vi "Straighten.vi"(6 "Go":bool, 8 "LockedHeading":dbl, 9 "Yaw":dbl, 10 "RightIn":dbl, 11 "LeftIn":dbl) -> (1 "Complete":bool, 2 "RightOut":dbl, 3 "LeftOut":dbl)   [LabVIEW 2015]
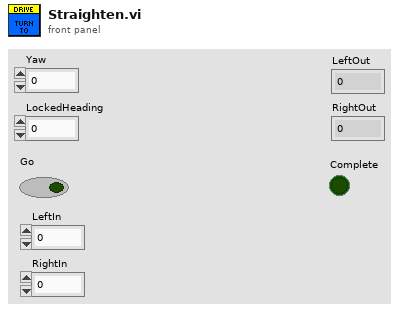
[diagram p1: front panel]
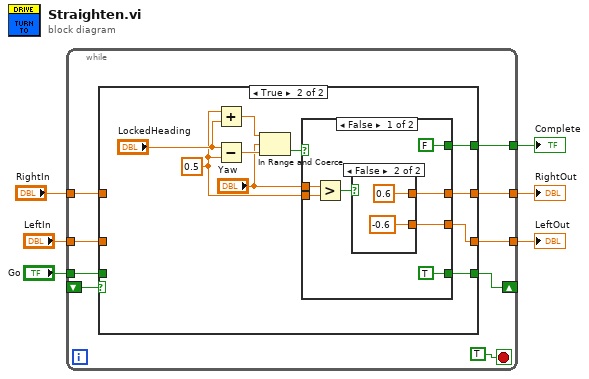
[diagram p0: block diagram]
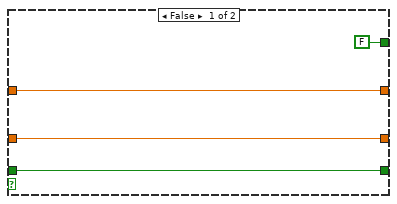
[diagram p2: hidden frame]
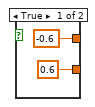
[diagram p3: hidden frame]
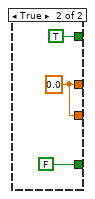
[diagram p4: hidden frame]
diagram:
  n1 = while {
    tunnel: "Go" -> [w15]
    shift-right: [w14] -> _
    shift-left: _ -> [w13]
    tunnel: "LeftIn" -> [w12]
    tunnel: [w11] -> w1
    tunnel: "RightIn" -> [w10]
    tunnel: [w9] -> w2
    tunnel: [w8] -> w3
    stop <- TRUE stop-if-true
    n2 = case shown="True" w13 {
      tunnel: [w19 w21] -> w14
      tunnel: w15 -> [w19 _]
      tunnel: [w18 w23] -> w11
      tunnel: w12 -> [w18 _]
      tunnel: [w17 w22] -> w9
      tunnel: w10 -> [w17 _]
      tunnel: [FALSE w20] -> w8
      frame False {
      }
      frame True {
        w25 = 0.5 ("y")
        n3 = Add(x=w25, y="LockedHeading") -> (x+y=w28:dbl)
        n4 = Subtract(x="LockedHeading", y=w25) -> (x-y=w27:dbl)
        n5 = In Range and Coerce(upper limit=w28, x="Yaw", lower limit=w27) -> (In Range?=w29:bool)  [unwired: 1 out]
        n6 = case shown="False" w29 {
          tunnel: w25 -> [w30 _]
          tunnel: "Yaw" -> [w31 _]
          tunnel: [w35 w43] -> w23
          tunnel: [w34 w43] -> w22
          tunnel: [TRUE FALSE] -> w21
          tunnel: [FALSE TRUE] -> w20
          frame False {
            n7 = Greater?(x=w31, y=w30) -> (0:w36:bool)
            n8 = case shown="False" w36 {
              tunnel: [0.6 -0.6] -> w35
              tunnel: [-0.6 0.6] -> w34
              frame True {
              }
              frame False {
              }
            }
          }
          frame True {
            w43 = 0.0
          }
        }
      }
    }
  }
  "LeftOut" <- w1
  "RightOut" <- w2
  "Complete" <- w3
